vi "Self Queue Alias.vi"(11 "Hello World Queue in":refnum<class "Hello World Queue.lvclass">) -> (2 "Self Queue Alias":string)   [LabVIEW 2021, in "Hello World Queue.lvlib" / "Hello World Queue.lvclass"]
uses:
  Hello World Queue.lvclass
  Hello World Queue.lvclass/Hello World Queue.ctl
  jettl/Queue jettl/Queue jettl.lvclass
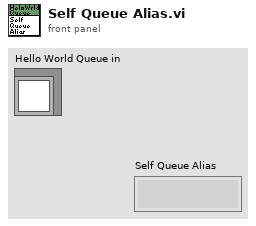
[diagram p1: front panel]
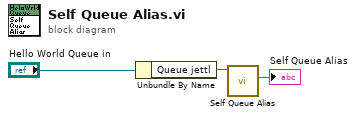
[diagram p0: block diagram]
diagram:
  n1 = Unbundle By Name("Hello World Queue in") -> ("Queue jettl"=w2:refnum<class "Queue jettl.lvclass">)
  n2 = call-dynamic "Self Queue Alias.vi"("Queue jettl in"=w2) -> ("Self Queue Alias"=→"Self Queue Alias":string)  [unwired: 10 in]
